vi "WriteConfig.vi"(8 "error in (no error)":errorcluster, 10 "Config":variant, 11 "PmuBase in":refnum<class "PmuBase.lvclass">) -> (0 "error out":errorcluster, 3 "PmuBase out":refnum<class "PmuBase.lvclass">)   [LabVIEW 2018, in "SensorPlugins.lvlib" / "PmuBase.lvclass"]
uses:
  PmuBase.lvclass
  Typedef/PmuConfig.ctl
  PmuBase.lvclass/PmuBase.ctl
  Accessors/Write PmuConfig.vi
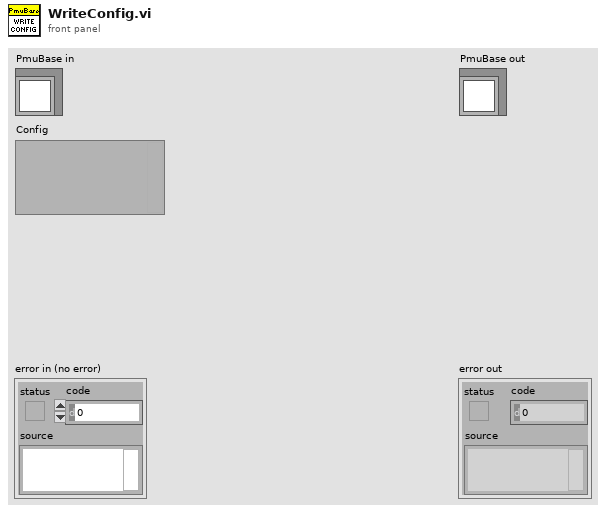
[diagram p1: front panel]
types:
  T1 = typedef "SensorPlugins.lvlib/PmuBase.lvclass/PmuConfig.ctl" = cluster{"Class":enum16{"M", "P"}, "Fs":i32, "F0":i32, "FSamp":i32, "SettlingTime":dbl, "T0":ext}
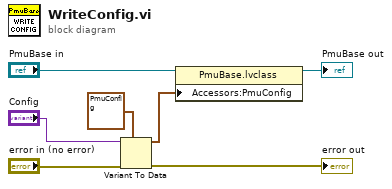
[diagram p0: block diagram]
diagram:
  n1 = Variant To Data(error in="error in (no error)", type=T1 {"Class"=enum."M", "Fs"=60, "F0"=60, "FSamp"=60, "SettlingTime"=0.0, "T0"=0.0} ("PmuConfig"), Variant="Config") -> (data=w3:T1, error out=→"error out":errorcluster)
  n2 = property class="PmuBase.lvclass"(reference="PmuBase in", "Accessors:PmuConfig"=w3) -> (reference out=→"PmuBase out":refnum<class "PmuBase.lvclass">)  [unwired: 1 in, 1 out]
